vi "AD5627R_Control.vi"(0 "RIO Device":T1, 1 "ADAPTER NAME":u8(ring) items=["1120 - 1 CH", "1212 - 2 CHs"], 2 "Vocm Offset(V)":dbl, 3 "error in (no error)":errorcluster, 4 "Selected Output":u8(ring) items=["Vout A", "Vout B"]) -> (5 "RIO Device out":T1, 6 "error out":errorcluster)   [LabVIEW 2018]
uses:
  <vilib>/userdefined/High Color/nirio_resource_hc.ctl
panel:
  in  "FSVocmDC":dbl=1.82
  in  "FSVocmDirect":dbl=1.05
  in  "Value":u16(knob) max=4095 scale=0.0..4095.0
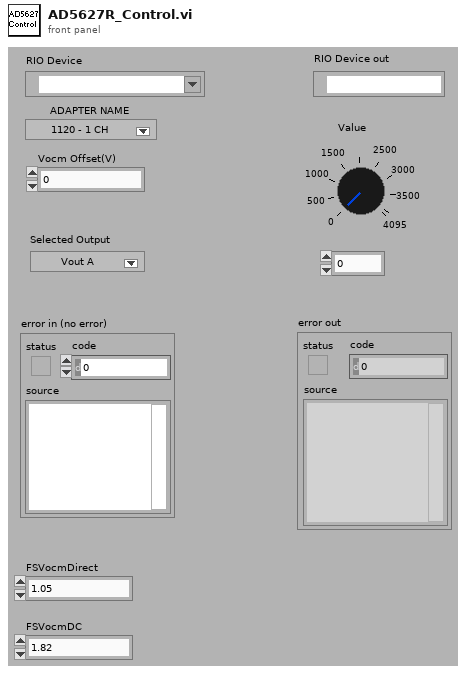
[diagram p1: front panel]
types:
  T1 = typedef "nirio_resource_hc.ctl" = tag
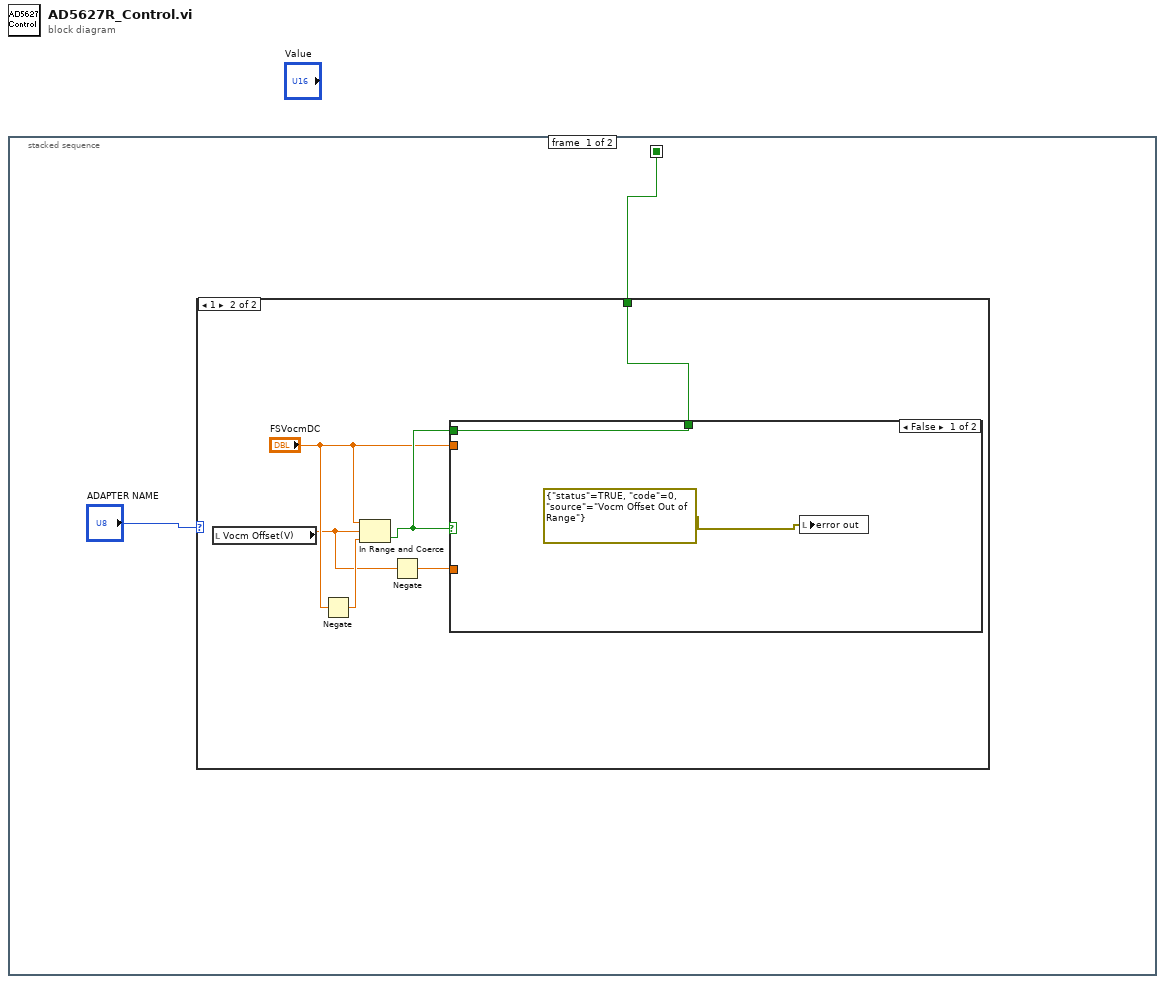
[diagram p0: block diagram]
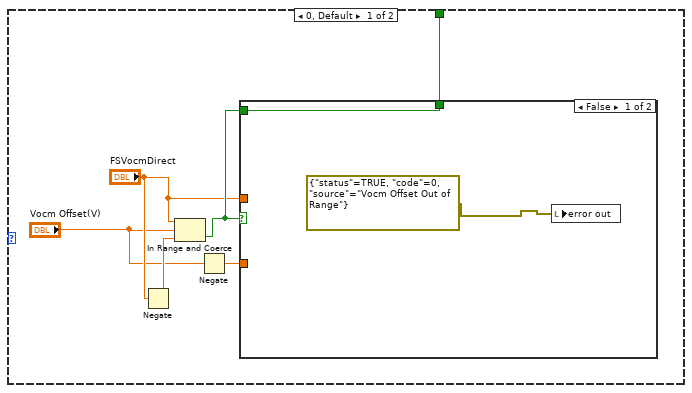
[diagram p2: hidden frame]
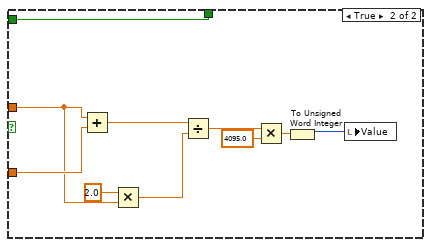
[diagram p3: hidden frame]
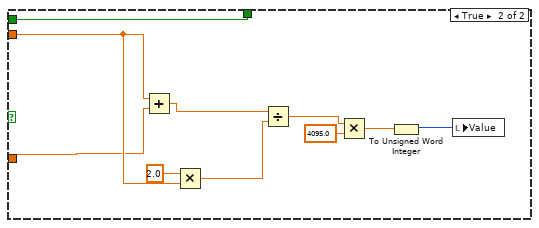
[diagram p4: hidden frame]
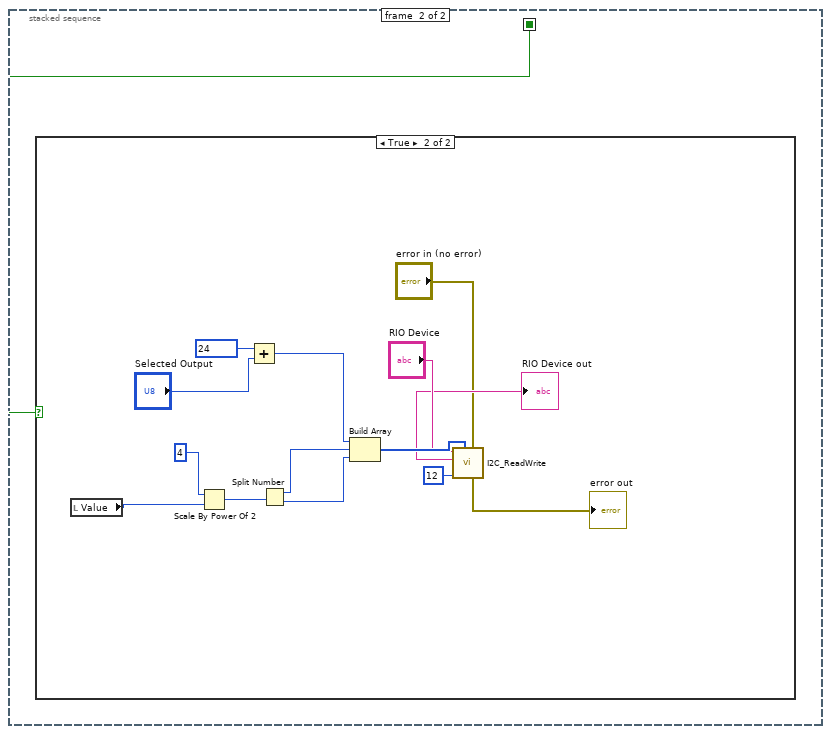
[diagram p5: hidden frame]
diagram:
  n1 = stacked-sequence {
    seq-local: [w1 _] -> [_ w39]
    frame #0 {
      n2 = case shown="1" "ADAPTER NAME" {
        tunnel: [w8 w26] -> w1
        frame 0, Default {
          n3 = Negate(x="FSVocmDirect") -> (-x=w6:dbl)
          n4 = In Range and Coerce(upper limit="FSVocmDirect", x="Vocm Offset(V)", lower limit=w6) -> (In Range?=w7:bool)  [unwired: 1 out]
          n5 = Negate(x="Vocm Offset(V)") -> (-x=w4:dbl)
          n6 = case shown="False" w7 {
            tunnel: [w10 w20] -> w8
            tunnel: w7 -> [w10 w20]
            tunnel: w4 -> [_ w19]
            tunnel: "FSVocmDirect" -> [_ w18]
            frame False {
              n7 = local write "error out"(errorcluster {"status"=TRUE, "code"=0, "source"="Vocm Offset Out of Range"} ("error out")) -> ()
            }
            frame True {
              n8 = Add(x=w18, y=w19) -> (x+y=w16:dbl)
              n9 = Multiply(x=2.0, y=w18) -> (x*y=w15:dbl)
              n10 = Divide(x=w16, y=w15) -> (x/y=w13:dbl)
              n11 = Multiply(x=w13, y=4095.0) -> (x*y=w12:dbl)
              n12 = To Unsigned Word Integer(number=w12) -> (unsigned 16bit integer=w11:u16)
              n13 = local write "Value"(w11) -> ()
            }
          }
        }
        frame 1 {
          n14 = local read "Vocm Offset(V)"() -> (w21:dbl)
          n15 = Negate(x="FSVocmDC") -> (-x=w23:dbl)
          n16 = In Range and Coerce(upper limit="FSVocmDC", x=w21, lower limit=w23) -> (In Range?=w25:bool)  [unwired: 1 out]
          n17 = Negate(x=w21) -> (-x=w22:dbl)
          n18 = case shown="False" w25 {
            tunnel: [w28 w38] -> w26
            tunnel: w25 -> [w28 w38]
            tunnel: "FSVocmDC" -> [_ w34]
            tunnel: w22 -> [_ w33]
            frame False {
              n19 = local write "error out"(errorcluster {"status"=TRUE, "code"=0, "source"="Vocm Offset Out of Range"} ("error out")) -> ()
            }
            frame True {
              n20 = Add(x=w34, y=w33) -> (x+y=w35:dbl)
              n21 = Multiply(x=2.0, y=w34) -> (x*y=w32:dbl)
              n22 = Divide(x=w35, y=w32) -> (x/y=w31:dbl)
              n23 = Multiply(x=w31, y=4095.0) -> (x*y=w30:dbl)
              n24 = To Unsigned Word Integer(number=w30) -> (unsigned 16bit integer=w29:u16)
              n25 = local write "Value"(w29) -> ()
            }
          }
        }
      }
    }
    frame #1 {
      n26 = case shown="True" w39 {
        frame False {
        }
        frame True {
          n27 = local read "Value"() -> (w40:u16)
          n28 = Scale By Power Of 2(n=u8 4 ("x"), x=w40) -> (x*2^n=w50:u16)
          n29 = Add(x=u8 24, y="Selected Output") -> (x+y=w51:u8)
          n30 = Split Number(x=w50) -> (hi(x)=w49:u8, lo(x)=w48:u8)
          n31 = Build Array(w51, w49, w48) -> (w45:u8[])
          n32 = call "I2C_ReadWrite.vi"("error in (no error)"="error in (no error)", "DataWriteArray"=w45, "Address"=u8 12, "RIO Device"="RIO Device") -> ("error out"=→"error out":errorcluster, "RIO Device out"=→"RIO Device out":T1)  [unwired: 5 in, 1 out]
        }
      }
    }
  }
